vi "Vision Research Phantom Series PhFile PhGetUseCase.vi"(0 "CH [in]":u64, 5 "Error In (no error)":errorcluster) -> (15 "pCineUseCaseID [out]":i32, 19 "Error Out":errorcluster)   [LabVIEW 2013, in "VRI.lvlib"]
doc: "PhGetUseCase\nHRESULT PhGetUseCase(CINEHANDLE CH, int* pCineUseCaseID);\n\nParameters\nCH [in]\n Cine to get the use case from.\npCineUseCaseID [out]\n Pointer where to store the use case.\n\nReturn Value\nThe function returns ERR_Ok in case of success or an error code, otherwise. To get extended error information call PhGetErrorMessage.\n\nRemarks\nReturns the current use case for the given cine.\n\nRequired Header\nPhFile.h"
uses:
  VRI.lvlib
  Phantom DLLs/PhFile.dll
panel:
  # "For instructions on the use of this VI, press Ctrl+H to display the help window and move the mouse over the icon, controls, and indicators"
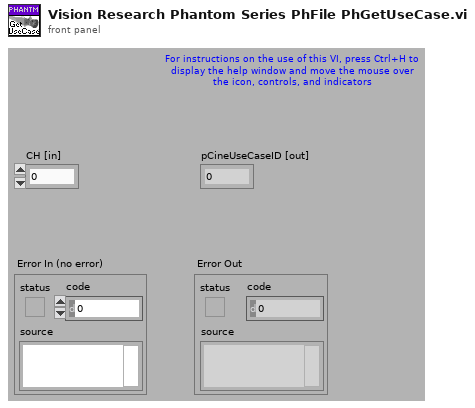
[diagram p1: front panel]
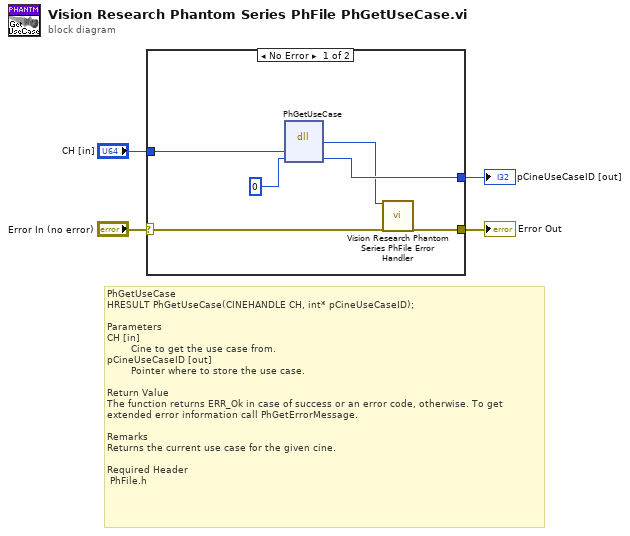
[diagram p0: block diagram]
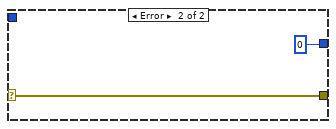
[diagram p2: hidden frame]
diagram:
  # "PhGetUseCase\nHRESULT PhGetUseCase(CINEHANDLE CH, int* pCineUseCaseID);\n\nParameters\nCH [in]\n        Cine to get the use case from.\npCineUseCaseID [out]\n        Pointer where to store the use case.\n\nReturn Value\nThe function returns ERR_Ok in case of success or an error code, otherwise. To get extended error information call PhGetErrorMessage.\n\nRemarks\nReturns the current use case for the given cine.\n\nRequired Header\n\tPhFile.h"
  n1 = case shown="No Error" "Error In (no error)" {
    selector: "Error In (no error)" -> [w10 w12]
    tunnel: [w9 w12] -> w3
    tunnel: "CH [in]" -> [w8 _]
    tunnel: [w7 0] -> w1
    frame No Error {
      n2 = dll-call lib="C:/Projects/SDK/32-bit/Vision Research Phantom Series Labview Driver/Phantom DLLs/PhFile.dll" fn="PhGetUseCase"("hC"=w8, "pCineUseCaseID"=0) -> ("HRESULT"=w5:i32, "pCineUseCaseID"=w7:i32)  [unwired: 4 in, 2 out]
      n3 = call "Vision Research Phantom Series PhFile Error Handler.vi"("Error Code (0)"=w5, "Error In (no error)"=w10) -> ("Error Out"=w9:errorcluster)  [unwired: 17 out]
    }
    frame Error {
    }
  }
  "Error Out" <- w3
  "pCineUseCaseID [out]" <- w1
